vi "read grid.vi"() -> ()   [LabVIEW 2022 SP3]
uses:
  Global 5 grid number.vi
panel:
  out "number":i32
  out "text":string
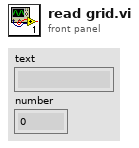
[diagram p1: front panel]
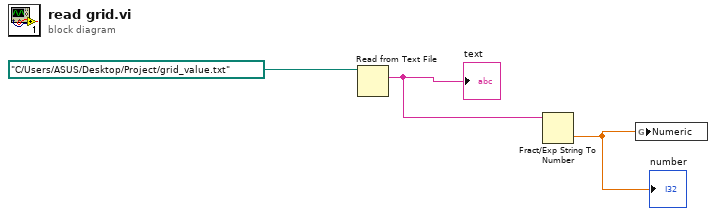
[diagram p0: block diagram]
diagram:
  n1 = Read from Text File(file (use dialog)=path "C:/Users/ASUS/Desktop/Project/grid_value.txt") -> (text=w2:string)  [unwired: 3 in, 3 out]
  "text" <- w2
  n2 = Fract/Exp String To Number(string=w2) -> (number=w1:dbl)  [unwired: 3 in, 1 out]
  "number" <- w1
  n3 = global write "Global 5 grid number.vi" "Numeric"(w1) -> ()
